vi "EV BMS Data Processed.vi"() -> ()   [LabVIEW 2017]
uses:
  <vilib>/addons/Electrical Power/EV Power Test/Battery/Power and Energy/NI_EP_Power and Energy.lvlib
  <vilib>/Analysis/2dsp.llb/Integral Method.ctl
  <vilib>/Analysis/NI_AALPro.lvlib
  <vilib>/addons/Electrical Power/EV Power Test/Battery/Power and Energy/Integrate Watt to Joule (1 Channel).vi
  <vilib>/addons/Electrical Power/EV Power Test/Battery/Power and Energy/Integrate Ampere to Coulomb (1 Channel).vi
  <vilib>/Waveform/WDTOps.llb/WDT Get Waveform Subset DBL.vi
panel:
  out "actual duration":dbl format="%0.2f"
  in  "file path":path
  out "Waveform Chart":T1(graph)
  out "battery pack data":T2(graph)
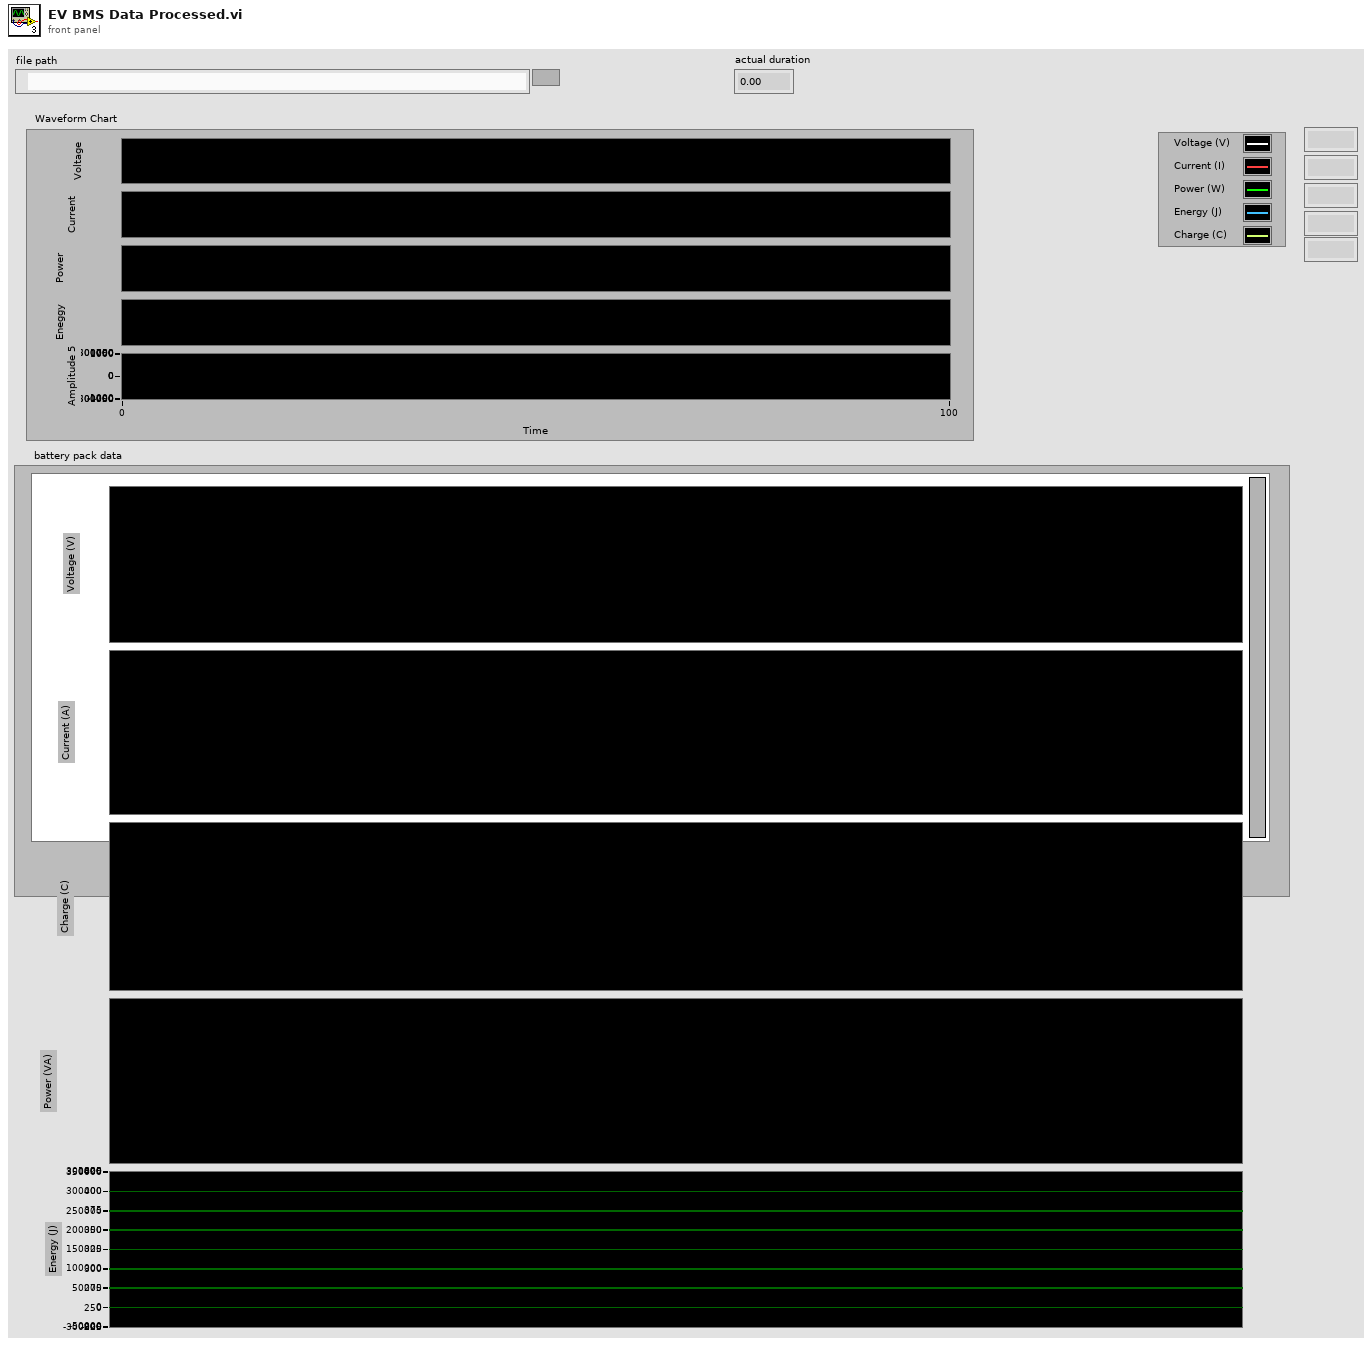
[diagram p1: front panel]
types:
  T1 = cluster{dbl, dbl, dbl, "cumulative energy [J]":dbl, "cumulative charge [C]":dbl}
  T2 = cluster{"PackVoltage":waveform(dbl), "PackCurrent":waveform(dbl), "PackCurrent":waveform(dbl), waveform(dbl), waveform(dbl)}
  T3 = cluster{dbl, dbl, dbl, "cumulative energy [J]":dbl, "cumulative charge [C]":dbl}[]
  T4 = enum16{"open", "open or create", "create or replace", "create", "open (read-only)"}
  T5 = typedef "NI_AALPro.lvlib/Integral Method.ctl" = i32
  T6 = cluster{waveform(dbl), waveform(dbl), waveform(dbl), waveform(dbl), waveform(dbl)}
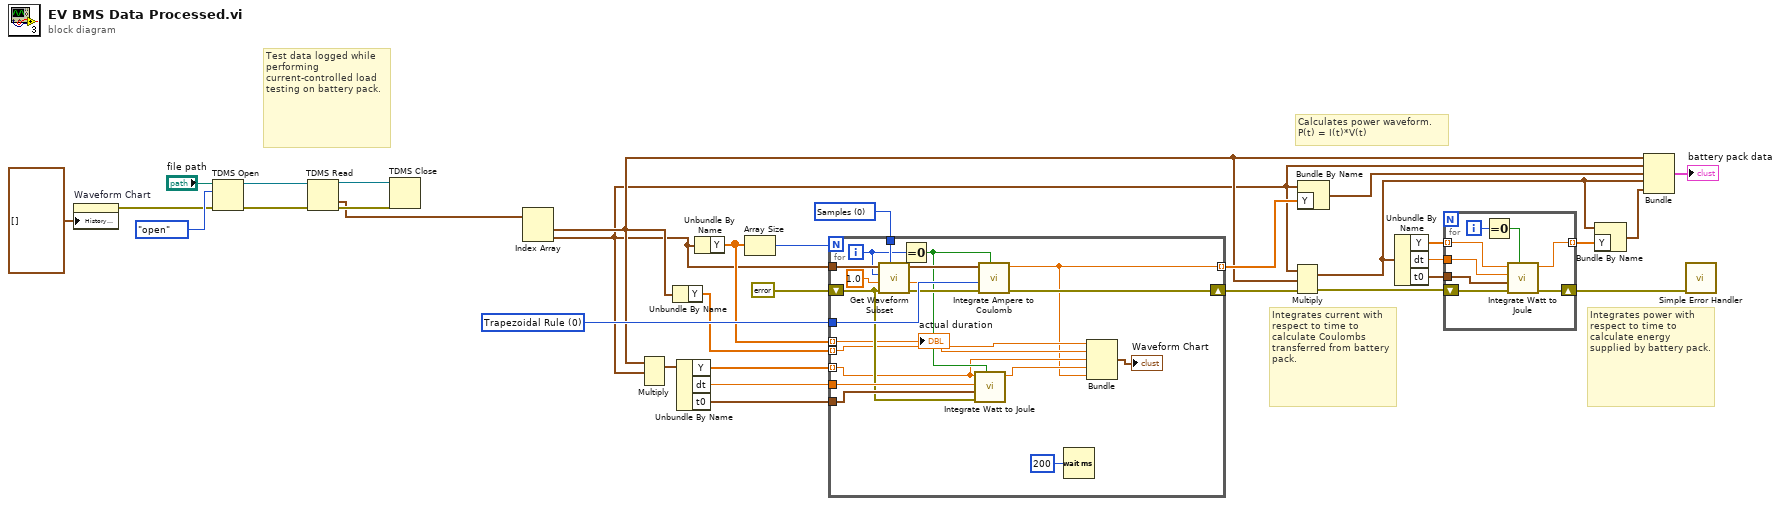
[diagram p0: block diagram]
diagram:
  w32 = T5 0 items=["Trapezoidal Rule", "Simpson's Rule", "Simpson's 3/8 Rule", "Bode Rule"] ("integration method")
  w33 = u16 0 items=["Samples", "Relative Time"] ("start/duration format")
  # "Calculates power waveform.\nP(t) = I(t)*V(t)"
  # "Test data logged while performing current-controlled load testing on battery pack."
  # "Integrates power with respect to time to calculate energy supplied by battery pack."
  # "Integrates current with respect to time to calculate Coulombs transferred from battery pack."
  n1 = property on="Waveform Chart" class="WFChart (strict)"("History Data"=T3 []) -> (error out=w1:errorcluster)  [unwired: 2 in, 1 out]
  n2 = TDMS Open(8:w1, 10:T4."open" ("operation (0:open)"), 11:"file path") -> (0:w9:errorcluster, 3:w11:refnum<k34>)  [unwired: 4 in]
  n3 = TDMS Read(0:w11, 11:w9) -> (4:w10:refnum<k34>, 10:w4:waveform(dbl)[], 15:w8:errorcluster)  [unwired: 6 in, 3 out]
  n4 = TDMS Close(8:w8, 11:w10) -> ()  [unwired: 2 out]
  n5 = Index Array(array=w4) -> (element #1=w3:waveform(dbl), element #2=w2:waveform(dbl))  [unwired: 2 in]
  n6 = Multiply(1:w2, 2:w3) -> (0:w17:waveform(dbl))  [unwired: 1 in, 1 out]
  n7 = Unbundle By Name(w3) -> ("Y"=w13:dbl[])
  n8 = Unbundle By Name(w17) -> ("Y"=w16:dbl[], "dt"=w15:dbl, "t0"=w14:timestamp)
  n9 = Unbundle By Name(w2) -> ("Y"=w12:dbl[])
  n10 = Array Size(array=w12) -> (size(s)=w30:i32)
  n11 = for {
    N: w30 -> [_]
    tunnel: w2 -> [w53]
    tunnel: w33 -> [w51]
    tunnel: w32 -> [w49]
    tunnel: [w37] -> w31 mode=indexing
    shift-right: [w47] -> w22
    shift-left: errorcluster {"status"=FALSE, "code"=0, "source"=""} ("no error") -> [w42]
    tunnel: w16 -> [w39] mode=indexing
    tunnel: w15 -> [w44]
    tunnel: w14 -> [w45]
    tunnel: w13 -> [w41] mode=indexing
    tunnel: w12 -> [w40] mode=indexing
    i -> [w46]
    n12 = call-poly <vilib>:"Get Waveform Subset.vi"("start/duration format"=w51, "error in (no error)"=w42, "duration"=1.0, "start samples/time"=w46, "waveform in"=w53) -> ("error out"=w48:errorcluster, "actual duration"=→"actual duration":dbl, "waveform out"=w52:waveform(dbl))  [unwired: 1 in, 1 out]
    n13 = Equal To 0?(x=w46) -> (x = 0?=w43:bool)
    n14 = call-poly <vilib>:"Integrate Watt to Joule.vi"("reset? (F)"=w43, "error in (no error)"=w42, "start timestamp"=w45, "interval duration [s]"=w44, "power [W]"=w39) -> ("cumulative energy [J]"=w38:dbl)  [unwired: 3 in, 3 out]
    n15 = call-poly <vilib>:"Integrate Ampere to Coulomb.vi"("reset? (F)"=w43, "error in (no error)"=w48, "integration method"=w49, "current waveform"=w52) -> ("error out"=w47:errorcluster, "cumulative charge [C]"=w37:dbl)  [unwired: 4 in, 2 out]
    n16 = Wait (ms)(milliseconds to wait=u32 200) -> ()  [unwired: 1 out]
    n17 = Bundle(w41, w40, w39, "cumulative energy [J]"=w38, "cumulative charge [C]"=w37) -> (→"Waveform Chart":T1)  [unwired: 1 in]
  }
  n18 = Multiply(1:w3, 2:w2, 4:w22) -> (0:w18:waveform(dbl), 3:w20:errorcluster)
  n19 = Bundle By Name(cluster=w2, "Y"=w31) -> (w24:waveform(dbl))
  n20 = Unbundle By Name(w18) -> ("Y"=w29:dbl[], "dt"=w28:dbl, "t0"=w27:timestamp)
  n21 = for {
    tunnel: w29 -> [w61] mode=indexing
    tunnel: w28 -> [w60]
    tunnel: w27 -> [w59]
    tunnel: [w56] -> w26 mode=indexing
    shift-right: [w54] -> w19
    shift-left: w20 -> [w55]
    i -> [w58]
    n22 = Equal To 0?(x=w58) -> (x = 0?=w57:bool)
    n23 = call-poly <vilib>:"Integrate Watt to Joule.vi"("reset? (F)"=w57, "error in (no error)"=w55, "start timestamp"=w59, "interval duration [s]"=w60, "power [W]"=w61) -> ("error out"=w54:errorcluster, "cumulative energy [J]"=w56:dbl)  [unwired: 3 in, 2 out]
  }
  n24 = Bundle By Name(cluster=w18, "Y"=w26) -> (w23:waveform(dbl))
  n25 = Bundle(w3, w2, w24, w18, w23) -> (→"battery pack data":T6)  [unwired: 1 in]
  n26 = call <vilib>:"Simple Error Handler.vi"("error in (no error)"=w19) -> ()  [unwired: 4 in, 5 out]
